vi "GetEventAllianceSelection.vi"(11 "Append to URL":string="CMP") -> (3 "value":T1)   [LabVIEW 2014, in "FIRST Events API.lvlib"]
uses:
  FIRST Events API.lvlib
  FRC Event Alliances.ctl
  FRC API Selector.ctl
panel:
  out "error out":errorcluster
  out "body":string
  out "headers":string
  out "Generated URL":string
  # "put \"CMP\" in for event"
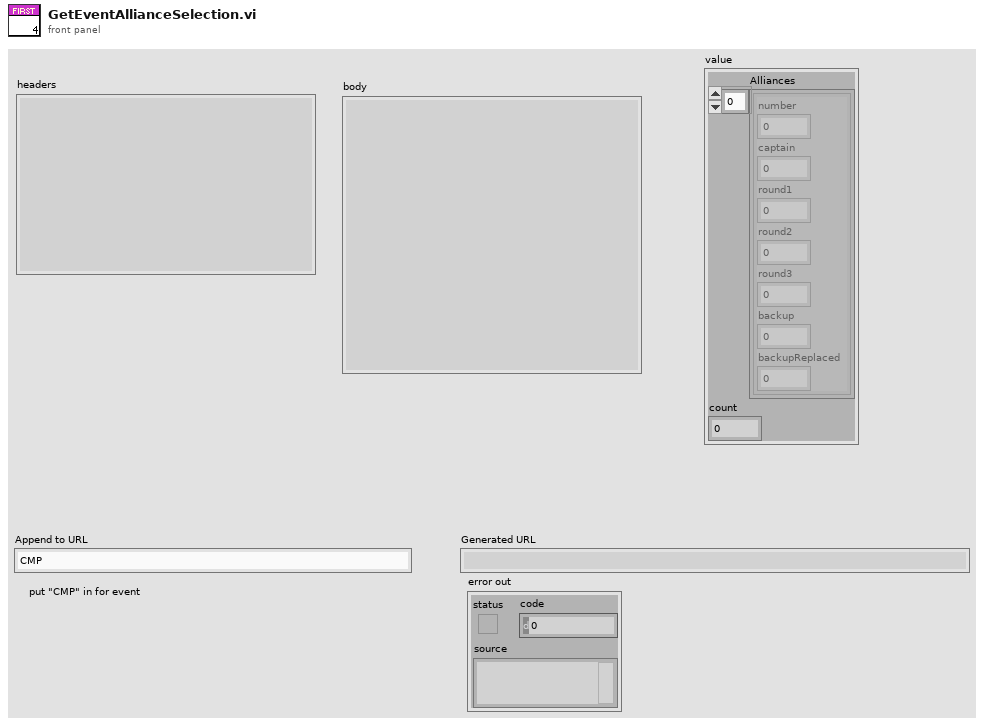
[diagram p1: front panel]
types:
  T1 = typedef "FIRST Events API.lvlib/FRC Event Alliances.ctl" = cluster{"Alliances":cluster{"number":i32, "captain":i32, "round1":i32, "round2":i32, "round3":i32, "backup":i32, "backupReplaced":i32}[], "count":i32}
  T2 = typedef "FIRST Events API.lvlib/FRC API Selector.ctl" = enum16{"GetEventAllianceSelection", "Ancillary", "GetTeamListings", "GetSchedule", "GetEventListings"}
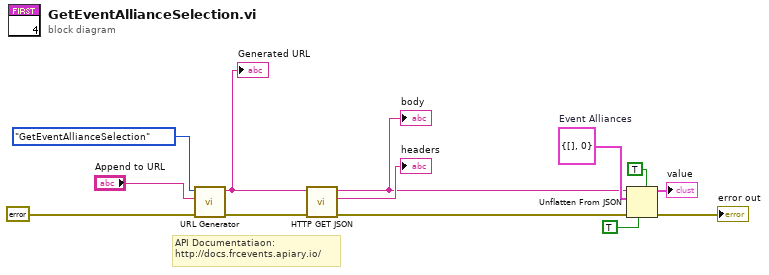
[diagram p0: block diagram]
diagram:
  w7 = T1 {"Alliances"=[], "count"=0}  # Event Alliances
  # "API Documentatiaon:\nhttp://docs.frcevents.apiary.io/"
  n1 = call "URL Generator.vi"("error in (no error)"=errorcluster {"status"=FALSE, "code"=0, "source"=""}, "Append URL"="Append to URL", "API Command"=FRC_API_Selector."GetEventAllianceSelection") -> ("error out"=w8:errorcluster, "Generated URL"=w11:string)  [unwired: 7 in]
  "Generated URL" <- w11
  n2 = call "HTTP GET JSON.vi"("error in (no error)"=w8, "Generated URL"=w11) -> ("error out"=w5:errorcluster, "headers"=→"headers":string, "body"=w6:string)  [unwired: 7 in]
  "body" <- w6
  n3 = Unflatten From JSON(enable LabVIEW extensions? (T)=TRUE, JSON string=w6, type and defaults=w7, default null elements? (F)=TRUE, error in (no error)=w5) -> (value=→"value":T1, error out=→"error out":errorcluster)  [unwired: 2 in]
